vi "HV ISet Single.vi"(9 "Current":string, 10 "Channel":string) -> (2 "Output":string)   [LabVIEW 2018, in "HV QMH.lvlib"]
uses:
  HV QMH.lvlib
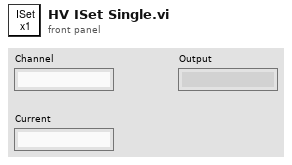
[diagram p1: front panel]
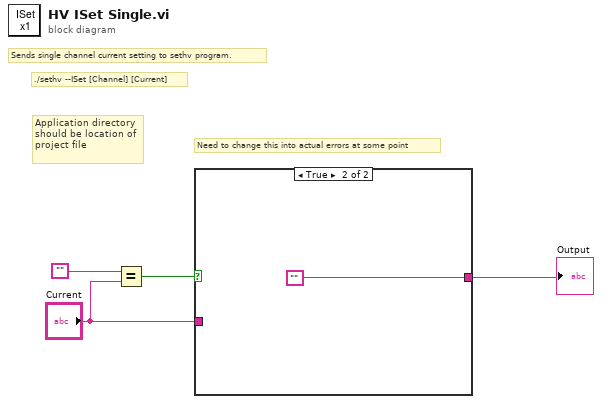
[diagram p0: block diagram]
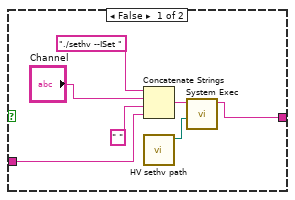
[diagram p2: hidden frame]
diagram:
  # "Need to change this into actual errors at some point"
  # "Application directory should be location of project file"
  # "Sends single channel current setting to sethv program."
  # "./sethv --ISet [Channel] [Current]"
  n1 = Equal?(x="", y="Current") -> (x = y?=w4:bool)
  n2 = case shown="True" w4 {
    tunnel: [w7 ""] -> w3
    tunnel: "Current" -> [w6 _]
    frame False {
      n3 = Concatenate Strings("./sethv --ISet ", "Channel", " ", w6) -> (w10:string)
      n4 = call "HV sethv path.vi"() -> ("sethv filepath"=w11:path)  [unwired: 11 in]
      n5 = call <vilib>:"System Exec.vi"("working directory"=w11, "command line"=w10) -> ("standard output"=w7:string)  [unwired: 6 in, 3 out]
    }
    frame True {
    }
  }
  "Output" <- w3
